vi "Set Camera Mode.vi"(8 "error in":errorcluster, 10 "Vision Mode":T2, 11 "VisionServerRef in":T1) -> (0 "error out":errorcluster, 3 "VisionServerRef out":T1)   [LabVIEW 2016, in "Vision Server.lvclass"]
uses:
  Vision Server.lvclass
  typedef/Vision Control Type.ctl
  typedef/Vision Server Ref.ctl
panel:
  # "Function not implemented on phone side..."
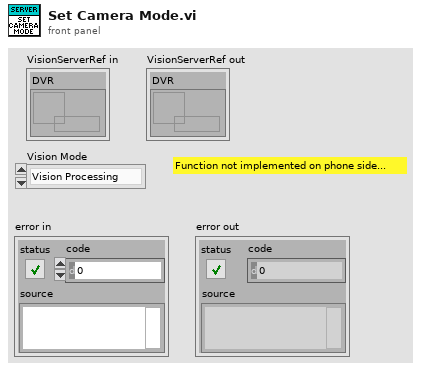
[diagram p1: front panel]
types:
  T1 = typedef "Vision Server.lvclass/Vision Server Ref.ctl" = cluster{"DVR":refnum<data-value>}
  T2 = typedef "Vision Server.lvclass/Vision Control Type.ctl" = enum16{"Vision Processing", "Driver Assistance"}
  T3 = typedef "Vision Server.lvclass/Message Type.ctl" = cluster{"type":string, "message":string}
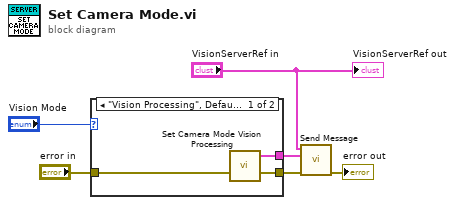
[diagram p0: block diagram]
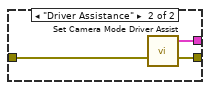
[diagram p2: hidden frame]
diagram:
  n1 = case shown="\"Vision Processing\", Default" "Vision Mode" {
    tunnel: "error in" -> [w8 w10]
    tunnel: [w8 w10] -> w4
    tunnel: [w7 w9] -> w2
    frame "Vision Processing", Default {
      n2 = call "Set Camera Mode Vision Processing.vi"() -> ("camera mode vision"=w7:T3)  [unwired: 2 in]
    }
    frame "Driver Assistance" {
      n3 = call "Set Camera Mode Driver Assist.vi"() -> ("camera mode vision"=w9:T3)  [unwired: 2 in]
    }
  }
  n4 = call "Send Message.vi"("error in"=w4, "Message"=w2, "VisionServerRef in"="VisionServerRef in") -> ("error out"=→"error out":errorcluster)  [unwired: 7 in, 1 out]
  "VisionServerRef out" <- "VisionServerRef in"
